vi "Create Helicopter Tasks.vi"(4 "Error In":errorcluster) -> (0 "Error Out":errorcluster, 3 "Hellicopter Tasks Output":T1)   [LabVIEW 2017]
uses:
  <vilib>/DAQmx/create/channels.llb/DAQmx Create Channel (AI-Voltage-Basic).vi
  <vilib>/DAQmx/configure/timing.llb/DAQmx Timing (Sample Clock).vi
  <vilib>/DAQmx/create/channels.llb/DAQmx Create Channel (CI-Position-Angular Encoder).vi
  <vilib>/DAQmx/create/channels.llb/DAQmx Create Channel (AO-Voltage-Basic).vi
  <vilib>/DAQmx/create/channels.llb/DAQmx Create Channel (DO-Digital Output).vi
  <resource>/objmgr/daqmx.rc
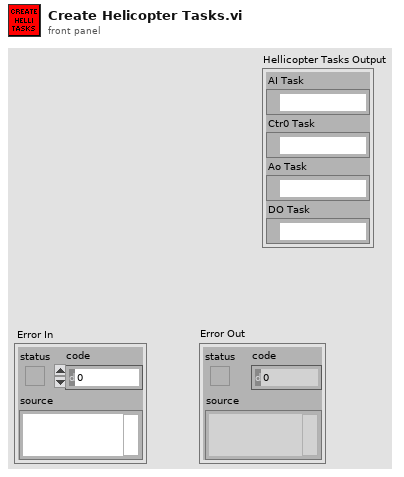
[diagram p1: front panel]
types:
  T1 = cluster{"AI Task":refnum<k21>, "Ctr0 Task":refnum<k21>, "Ao Task":refnum<k21>, "DO Task":refnum<k21>}
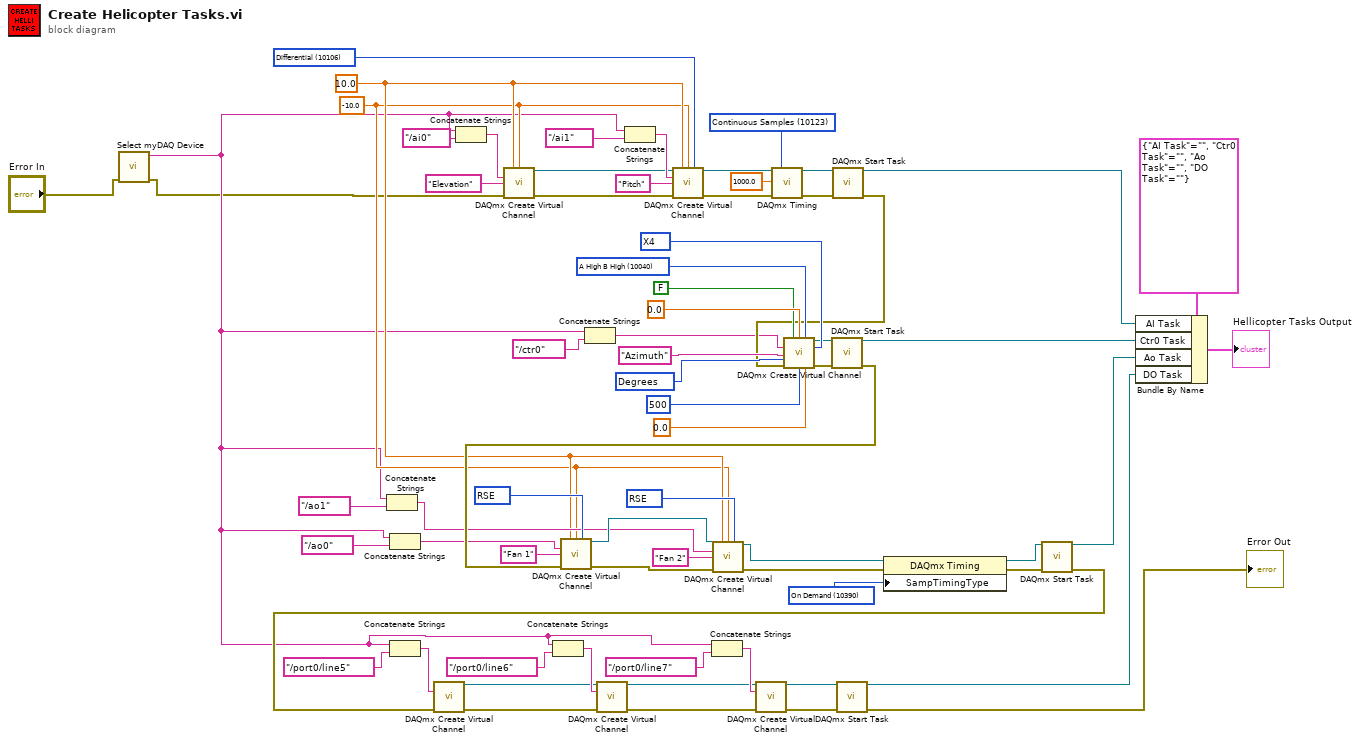
[diagram p0: block diagram]
diagram:
  w8 = 10390 items=["Sample Clock"=10388, "Burst Handshake"=12548, "Handshake"=10389, "Implicit"=10451, "On Demand"=10390, "Change Detection"=12504, "Pipelined Sample Clock"=14668] ("SampTimingType")
  w69 = 10083 items=["Default"=-1, "RSE"=10083, "Differential"=10106, "Pseudodifferential"=12529] ("output terminal configuration")
  w64 = 10083 items=["Default"=-1, "RSE"=10083, "Differential"=10106, "Pseudodifferential"=12529] ("output terminal configuration")
  w61 = 10146 items=["Degrees"=10146, "Radians"=10273, "Ticks"=10304, "From Custom Scale"=10065] ("units")
  w58 = 10040 items=["A High B High"=10040, "A High B Low"=10041, "A Low B High"=10042, "A Low B Low"=10043] ("z index phase")
  w57 = 10092 items=["X1"=10090, "X2"=10091, "X4"=10092, "Two Pulse Counting"=10313] ("decoding type")
  w51 = 10123 items=["Finite Samples"=10178, "Continuous Samples"=10123, "Hardware Timed Single Point"=12522] ("sample mode")
  w47 = 10106 items=["default"=-1, "RSE"=10083, "NRSE"=10078, "Differential"=10106, "Pseudodifferential"=12529] ("input terminal configuration")
  w11 = -10.0 ("minimum value")
  w12 = 10.0 ("maximum value")
  n1 = call "Select myDAQ Device.vi"("Error In"="Error In") -> ("Error Out"=w2:errorcluster, "DAQmx Device Name"=w3:tag)  [unwired: 9 in]
  n2 = Concatenate Strings(w3, tag "/ao1" ("physical channels")) -> (w34:string)
  n3 = Concatenate Strings(w3, tag "/ao0" ("physical channels")) -> (w35:string)
  n4 = Concatenate Strings(w3, tag "/port0/line5" ("lines")) -> (w30:string)
  n5 = Concatenate Strings(w3, tag "/ai0" ("physical channels")) -> (w16:string)
  n6 = call-poly <vilib>:"DAQmx Create Virtual Channel.vi"("maximum value"=w12, "minimum value"=w11, "physical channels"=w16, "name to assign"="Elevation", "error in"=w2) -> ("task out"=w13:refnum<k21>, "error out"=w10:errorcluster)  [unwired: 9 in]
  n7 = Concatenate Strings(w3, tag "/port0/line6" ("lines")) -> (w29:string)
  n8 = Concatenate Strings(w3, tag "/ctr0" ("counter")) -> (w38:string)
  n9 = Concatenate Strings(w3, tag "/ai1" ("physical channels")) -> (w32:string)
  n10 = call-poly <vilib>:"DAQmx Create Virtual Channel.vi"("task in"=w13, "maximum value"=w12, "minimum value"=w11, "input terminal configuration"=w47, "physical channels"=w32, "name to assign"="Pitch", "error in"=w10) -> ("task out"=w48:refnum<k21>, "error out"=w49:errorcluster)  [unwired: 7 in]
  n11 = Concatenate Strings(w3, tag "/port0/line7" ("lines")) -> (w28:string)
  n12 = call-poly <vilib>:"DAQmx Timing.vi"("task/channels in"=w48, "sample mode"=w51, "rate"=1000.0, "error in"=w49) -> ("task out"=w52:refnum<k21>, "error out"=w55:errorcluster)  [unwired: 10 in]
  n13 = call <vilib>:"DAQmx Start Task.vi"("task/channels in"=w52, "error in"=w55) -> ("task out"=w42:refnum<k21>, "error out"=w45:errorcluster)  [unwired: 12 in]
  n14 = call-poly <vilib>:"DAQmx Create Virtual Channel.vi"("z index enable"=FALSE, "z index value"=0.0, "z index phase"=w58, "counter"=w38, "decoding type"=w57, "name to assign"="Azimuth", "units"=w61, "error in"=w45, "pulses per revolution"=u32 500, "initial angle"=0.0) -> ("task out"=w56:refnum<k21>, "error out"=w60:errorcluster)  [unwired: 4 in]
  n15 = call <vilib>:"DAQmx Start Task.vi"("task/channels in"=w56, "error in"=w60) -> ("task out"=w41:refnum<k21>, "error out"=w44:errorcluster)  [unwired: 12 in]
  n16 = call-poly <vilib>:"DAQmx Create Virtual Channel.vi"("maximum value"=w12, "minimum value"=w11, "output terminal configuration"=w69, "physical channels"=w35, "name to assign"="Fan 1", "error in"=w44) -> ("task out"=w67:refnum<k21>, "error out"=w68:errorcluster)  [unwired: 8 in]
  n17 = call-poly <vilib>:"DAQmx Create Virtual Channel.vi"("task in"=w67, "maximum value"=w12, "minimum value"=w11, "output terminal configuration"=w64, "physical channels"=w34, "name to assign"="Fan 2", "error in"=w68) -> ("task out"=w5:refnum<k21>, "error out"=w4:errorcluster)  [unwired: 7 in]
  n18 = property class="DAQmx Timing"(reference=w5, error in=w4, "SampTimingType"=w8) -> (reference out=w6:refnum<k21>, error out=w7:errorcluster)
  n19 = call <vilib>:"DAQmx Start Task.vi"("task/channels in"=w6, "error in"=w7) -> ("task out"=w40:refnum<k21>, "error out"=w21:errorcluster)  [unwired: 12 in]
  n20 = call-poly <vilib>:"DAQmx Create Virtual Channel.vi"("lines"=w30, "error in"=w21) -> ("task out"=w25:refnum<k21>, "error out"=w22:errorcluster)  [unwired: 12 in]
  n21 = call-poly <vilib>:"DAQmx Create Virtual Channel.vi"("task in"=w25, "lines"=w29, "error in"=w22) -> ("task out"=w24:refnum<k21>, "error out"=w23:errorcluster)  [unwired: 11 in]
  n22 = call-poly <vilib>:"DAQmx Create Virtual Channel.vi"("task in"=w24, "lines"=w28, "error in"=w23) -> ("task out"=w18:refnum<k21>, "error out"=w20:errorcluster)  [unwired: 11 in]
  n23 = call <vilib>:"DAQmx Start Task.vi"("task/channels in"=w18, "error in"=w20) -> ("task out"=w17:refnum<k21>, "error out"=→"Error Out":errorcluster)  [unwired: 12 in]
  n24 = Bundle By Name(cluster=T1 {"AI Task"="", "Ctr0 Task"="", "Ao Task"="", "DO Task"=""}, "AI Task"=w42, "Ctr0 Task"=w41, "Ao Task"=w40, "DO Task"=w17) -> (→"Hellicopter Tasks Output":T1)
